vi "tstp_can_request_and_get_response.vi"(8 "错误输入（无错误）":errorcluster, 9 "AReqDataArray":u8[](array[numeric]), 10 "ADiagModuleIndex":i32, 11 "path":path) -> (0 "错误输出":errorcluster, 1 "Diagnostic response":u8[](array[numeric]), 2 "Return Type":i32, 3 "path out":path)   [LabVIEW 2014]
doc: "Function Introduction :\nRequest ID to request data and obtain response data\nCall location :\ninput parameter :\nADiagModulus Index: Handle to UDS module\nAReqDataArray: A data pointer pointing to the requested data source\nAReqDataSize: The size of the data source array in bytes\nAResponseDataArray: a data pointer pointing to the response data buffer\nAResponseDataSize: A data pointer pointing to an integer value, used to store the size of the response data\nReturn value :\n==0: Execution successful\nOther values: Query error code"
panel:
  in  "Cluster":T1
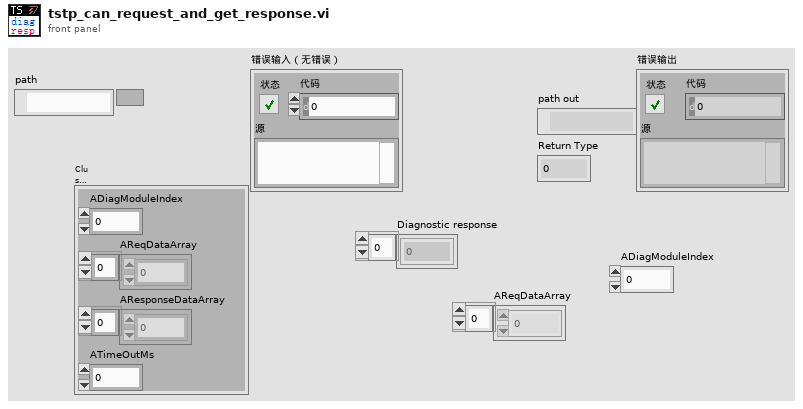
[diagram p1: front panel]
types:
  T1 = cluster{"ADiagModuleIndex":i32, "AReqDataArray":u8[], "AResponseDataArray":u8[], "ATimeOutMs":i32}
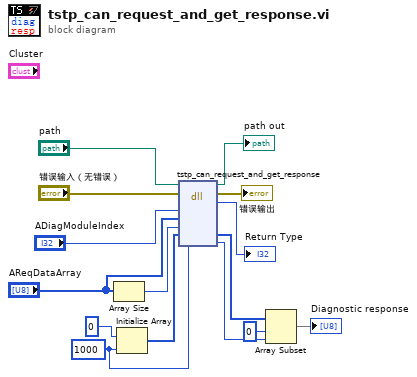
[diagram p0: block diagram]
diagram:
  w3 = 1000 ("dimension size")
  n1 = Array Size(array="AReqDataArray") -> (size(s)=w4:i32)
  n2 = Initialize Array(u8 0, w3) -> (w7:u8[])
  n3 = dll-call lib="C:/Users/XYY/Desktop/LabView Demo/TSCAN_LB2018_V1.3_20220301/Config/TSMaster.dll" fn="tstp_can_request_and_get_response"(path in="path", error in="错误输入（无错误）", "ADiagModuleIndex"="ADiagModuleIndex", "AReqDataArray"="AReqDataArray", "AReqDataSize"=w4, "AResponseDataArray"=w7, "AResponseDataSize"=w3) -> (path out=→"path out":path, error out=→"错误输出":errorcluster, "返回类型"=→"Return Type":i32, "AResponseDataArray"=w6:u8[], "AResponseDataSize"=w2:i32)  [unwired: 4 in]
  n4 = Array Subset(array=w6, index=0 ("索引"), length=w2) -> (→"Diagnostic response":u8[])
